vi "Resample VR Data.vi"(7 "Memory Size":i32=32768, 11 "Data In":dbl[](array[numeric])) -> (3 "Resampled Data":dbl[](array[numeric]))   [LabVIEW 2013, in "Engine Simulation Toolkit System Explorer.lvlib"]
uses:
  Engine Simulation Toolkit System Explorer.lvlib
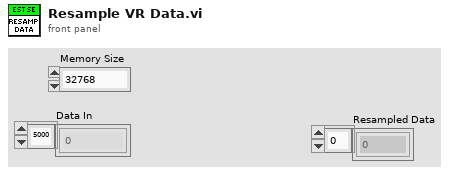
[diagram p1: front panel]
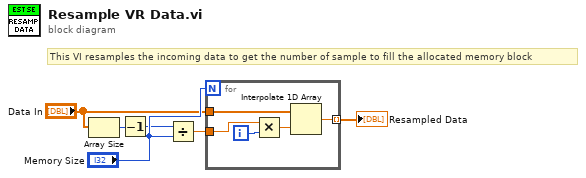
[diagram p0: block diagram]
diagram:
  # "This VI resamples the incoming data to get the number of sample to fill the allocated memory block"
  n1 = Array Size(array="Data In") -> (size(s)=w6:i32)
  n2 = Decrement(x=w6) -> (x-1=w1:i32)
  n3 = Divide(x=w1, y="Memory Size") -> (x/y=w5:dbl)
  n4 = for {
    N: "Memory Size" -> [_]
    tunnel: "Data In" -> [w11]
    tunnel: [w10] -> w3 mode=indexing
    tunnel: w5 -> [w8]
    i -> [w9]
    n5 = Multiply(x=w8, y=w9) -> (x*y=w7:dbl)
    n6 = Interpolate 1D Array(1:w7, 2:w11) -> (0:w10:dbl)
  }
  "Resampled Data" <- w3
